vi "Open VISA.vi"(8 "错误输入（无错误）":errorcluster, 11 "VISA":T1={"VISA"="", "baud rate"=9600, "data bits"=8, "parity"=enum."None", "stop bits"=10, "flow control"=0} {"flow control" items=["None", "XON/XOFF", "RTS/CTS", "XON/XOFF & RTS/CTS", "DTR/DSR", "XON/XOFF & DTR/DSR"]; "stop bits" items=["1.0"=10, "1.5"=15, "2.0"=20]}) -> (0 "error out":errorcluster caption="错误输出", 3 "VISA resource name out":refnum<visa-resource-name> caption="VISA资源名称输出")   [LabVIEW 2014]
uses:
  <vilib>/Instr/_visa.llb/VISA Configure Serial Port (Instr).vi
  Ctr/VISA Ctr.ctl
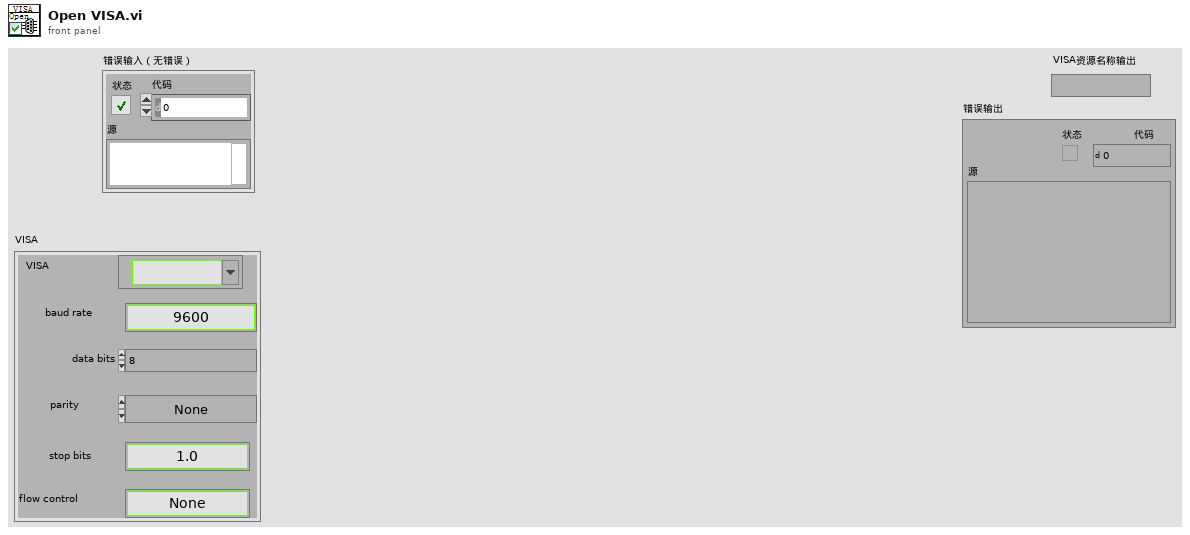
[diagram p1: front panel]
types:
  T1 = typedef "VISA Ctr.ctl" = cluster{"VISA":refnum<visa-resource-name>, "baud rate":u32, "data bits":u16, "parity":enum16{"None", "Odd", "Even", "Mark", "Space"}, "stop bits":u16, "flow control":u16}
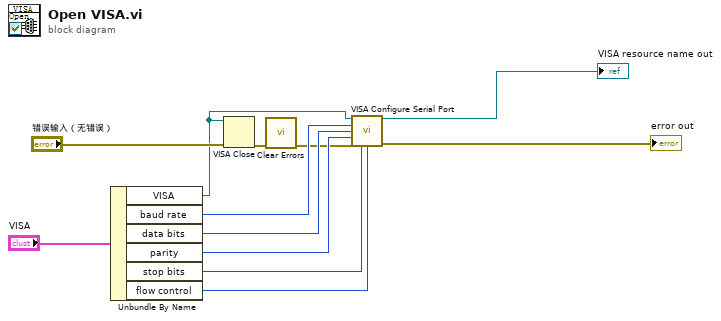
[diagram p0: block diagram]
diagram:
  n1 = Unbundle By Name("VISA") -> ("VISA"=w5:refnum<visa-resource-name>, "baud rate"=w11:u32, "data bits"=w10:u16, "parity"=w9:enum16{"None", "Odd", "Even", "Mark", "Space"}, "stop bits"=w8:u16, "flow control"=w7:u16)
  n2 = VISA Close(VISA resource name=w5, error in (no error)="错误输入（无错误）") -> (error out=w2:errorcluster)
  n3 = call <vilib>:"Clear Errors.vi"("error in (no error)"=w2) -> ("error out"=w1:errorcluster)  [unwired: 5 in, 1 out]
  n4 = call-poly "VISA Configure Serial Port"("VISA resource name"=w5, "baud rate (9600)"=w11, "data bits (8)"=w10, "parity (0:none)"=w9, "error in (no error)"=w1, "stop bits (10: 1 bit)"=w8, "flow control (0:none)"=w7) -> ("VISA resource name out"=→"VISA resource name out":refnum<visa-resource-name>, "error out"=→"error out":errorcluster)  [unwired: 7 in]
